vi "sit IO cRIO9113.vi"() -> ()   [LabVIEW 2010]
uses:
  <vilib>/Platform/TimedLoop/XDataNode/XDataNode.xnode
  <vilib>/Platform/TimedLoop/XDataNode/timing_clust.ctl
  <vilib>/Platform/TimedLoop/XDataNode/nitl_modes.ctl
  <vilib>/Platform/TimedLoop/XDataNode/wakeup.ctl
  <vilib>/eio/EIONode/EIONode.xnode
  <vilib>/rvi/eio/nirviEIOImplementation/nirviEIOImplementation.xnode
  <vilib>/rvi/eio/common/nirviEmuClasses.ctl
  <vilib>/rvi/Arithmetic/AddSubMult/XNode/nirviSatArithmetic.xnode
  <vilib>/rvi/eio/common/nirviEmuTemplateMethod_noerrors.vi
  <vilib>/Platform/TimedLoop/XDataNode/XDNodeRunTimeDep.lvlib
panel:
  in  "Velocity Interval (uSec)":u32=200000
  out "Velocity (Counts/Interval)":i32
  out "Acceleration (Counts/Interval)":i32
  out "Position (Counts)":i32
  in  "Position Reset 2":bool
  out "Rudder (Counts)":i32
  in  "Rudder Position Reset":bool
  in  "PWM out 2 (DO 6)":u32[](array[numeric])=[0, 0]
  in  "PWM out 3 (DO 7)":u32[](array[numeric])=[0, 0]
  in  "_PWM In 1 timeout":u32=40000
  out "_PWM In 1 High Time":u32
  out "_PWM In 1 Low Time":u32
  out "_PWM In 0 Low Time":u32
  out "_PWM In 0 High Time":u32
  in  "_PWM In 0 timeout":u32=40000
  in  "_Low Pulse 1":u32
  in  "_High Pulse 1":u32
  in  "_Low Pulse 3":u32
  in  "_High Pulse 3":u32
  in  "_Low Pulse 2":u32
  in  "_High Pulse 2":u32
  in  "PWM out 0 (DO 4)":u32[](array[numeric])=[0, 0]
  in  "PWM out 1 (DO 5)":u32[](array[numeric])=[0, 0]
  out "PWM in 1 (DI 5)":u32[](array[numeric])
  out "PWM in 0 (DI 4)":u32[](array[numeric])
  in  "_Low Pulse 0":u32
  in  "_High Pulse 0":u32
  in  "DO 0":bool
  in  "DO 1":bool
  in  "DO 2":bool
  in  "DO 3":bool
  out "DI 4":bool
  out "DI 5":bool
  in  "Reset":bool
  out "Late? Latched":bool
  in  "Wait Until Cleared":bool=TRUE
  in  "Local Stop 0":bool
  in  "Start 0":bool
  in  "_IRQ bit (0-31)":u8
  in  "Loop Rate (usec)":u32=300
  # "Configuration"
  # "Encoders"
  # "Digital"
  # "PWM"
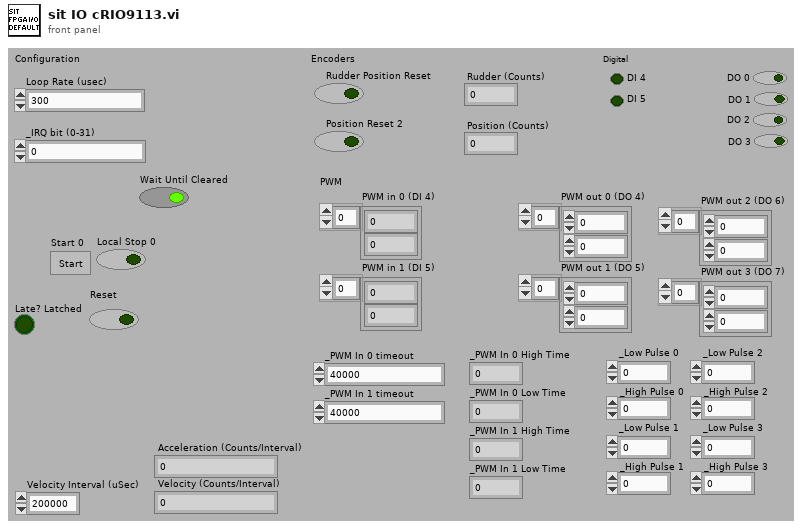
[diagram p1: front panel]
types:
  T1 = typedef "XDNodeRunTimeDep.lvlib/timing_clust.ctl" = cluster{"Expected End [f-1]":u64, "Actual End [f-1]":u64, "Finished Late? [f-1]":bool, "Expected End [i-1]":u64, "Actual End [i-1]":u64, "Finished Late? [i-1]":bool, "Expected Start [i]":u64, "Actual Start [i]":u64, "Expected Start [f]":u64, "Actual Start [f]":u64, "Source Name":string, "Structure Name":string, "Period":i64, "Deadline":i64, "Offset":i64, "Start":i64, "Priority":i32, "Timeout":i32, "Mode":T2, "Wakeup Reason":T3, "Error":errorcluster, "Source Type":string, "Secondary Source Type":string, "Global End Time":u64, "Global Start Time":u64, "Frame Duration":u64, "Iteration Duration":u64, "Assigned CPU":i32, "I/O Scan Engine Mode":u32}
  T2 = typedef "XDNodeRunTimeDep.lvlib/nitl_modes.ctl" = enum32{"No Change", "Process missed periods, maintain original phase", "Discard missed periods, maintain original phase", "Process missed periods, ignore original phase", "Discard missed periods, ignore original phase"}
  T3 = typedef "XDNodeRunTimeDep.lvlib/wakeup.ctl" = enum32{"Normal", "Aborted", "Asynchronous wakeup", "Timing source error", "Timed loop error", "Timeout"}
  T4 = typedef "nirviEmuClasses.ctl" = enum16{"IO Read", "IO Write", "Method", "Property Read", "Property Write"}
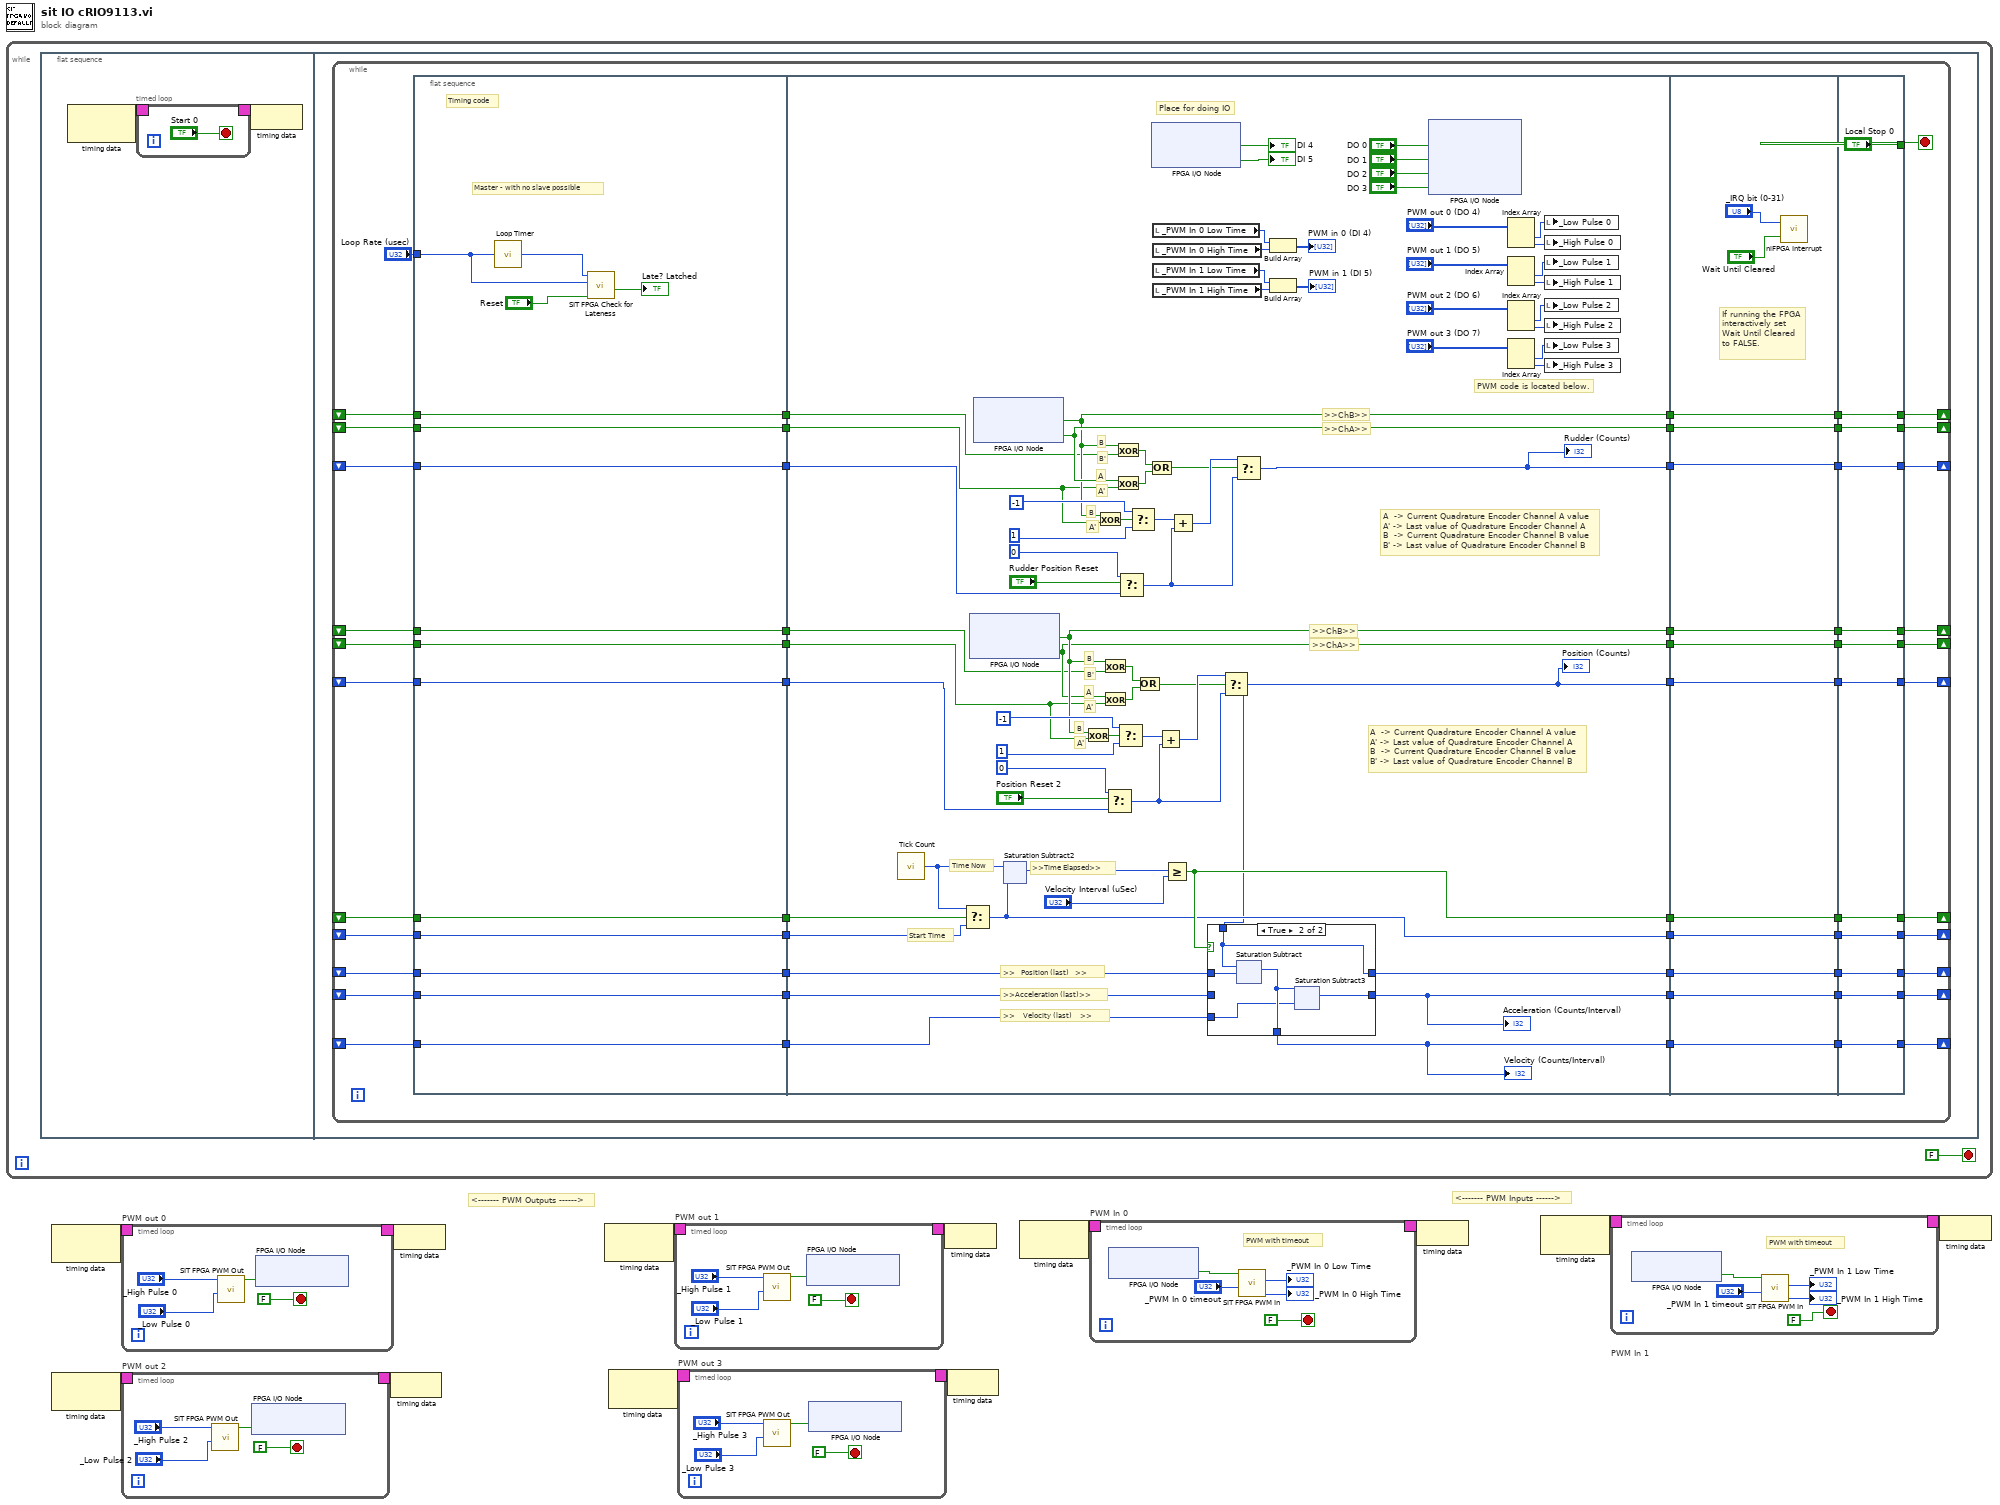
[diagram p0: block diagram]
diagram:
  # "<------- PWM Outputs ------>"
  # "<------- PWM Inputs ------>"
  n1 = while {
    stop <- FALSE stop-if-true
    n2 = flat-sequence {
      frame #0 {
        n3 = node-c288 ("Input Node")() -> (w15:T1)  [unwired: 1 out]
        n4 = timed-loop "initWait" {
          timing: w15 -> [_]
          timing-out: [_] -> w14
          stop <- "Start 0" stop-if-true
        }
        n5 = node-c288 ("Output Node")(w14) -> ()
      }
      frame #1 {
        n6 = while {
          shift-right: [w72] -> _
          shift-left: _ -> [w65]
          shift-right: [w73] -> _
          shift-left: _ -> [w63]
          shift-right: [w69] -> _
          shift-left: _ -> [w61]
          shift-right: [w60] -> _
          shift-left: _ -> [w50]
          shift-right: [w57] -> _
          shift-left: _ -> [w48]
          shift-right: [w54] -> _
          shift-left: _ -> [w46]
          shift-right: [w45] -> _
          shift-left: _ -> [w29]
          shift-right: [w39] -> _
          shift-left: _ -> [w25]
          shift-right: [w42] -> _
          shift-left: _ -> [w27]
          shift-right: [w36] -> _
          shift-left: _ -> [w23]
          shift-right: [w33] -> _
          shift-left: _ -> [w21]
          stop <- w76 stop-if-true
          n7 = flat-sequence {
            tunnel: "Loop Rate (usec)" -> [w78]
            tunnel: [w89] -> w66
            tunnel: w65 -> [w89]
            tunnel: [w88] -> w64
            tunnel: w63 -> [w88]
            tunnel: [w87] -> w62
            tunnel: w61 -> [w87]
            tunnel: [w86] -> w51
            tunnel: w50 -> [w86]
            tunnel: [w85] -> w49
            tunnel: w48 -> [w85]
            tunnel: [w84] -> w47
            tunnel: w46 -> [w84]
            tunnel: [w83] -> w30
            tunnel: w29 -> [w83]
            tunnel: [w82] -> w28
            tunnel: w27 -> [w82]
            tunnel: [w81] -> w26
            tunnel: w25 -> [w81]
            tunnel: [w80] -> w24
            tunnel: w23 -> [w80]
            tunnel: [w79] -> w22
            tunnel: w21 -> [w79]
            tunnel: [w128] -> w74
            tunnel: [w127] -> w70
            tunnel: [w97] -> w67
            tunnel: w66 -> [w126]
            tunnel: w64 -> [w125]
            tunnel: w62 -> [w124]
            tunnel: [w112] -> w58
            tunnel: [w111] -> w55
            tunnel: [w96] -> w52
            tunnel: w51 -> [w110]
            tunnel: w49 -> [w109]
            tunnel: w47 -> [w108]
            tunnel: [w105] -> w43
            tunnel: [w104] -> w40
            tunnel: [w103] -> w37
            tunnel: [w94] -> w34
            tunnel: [w93] -> w31
            tunnel: w30 -> [w102]
            tunnel: w28 -> [w101]
            tunnel: w26 -> [w100]
            tunnel: w24 -> [w99]
            tunnel: w22 -> [w98]
            tunnel: [w386] -> w75
            tunnel: w74 -> [w386]
            tunnel: [w385] -> w71
            tunnel: w70 -> [w385]
            tunnel: [w384] -> w68
            tunnel: w67 -> [w384]
            tunnel: [w383] -> w59
            tunnel: w58 -> [w383]
            tunnel: [w382] -> w56
            tunnel: w55 -> [w382]
            tunnel: [w381] -> w53
            tunnel: w52 -> [w381]
            tunnel: [w380] -> w44
            tunnel: w43 -> [w380]
            tunnel: [w379] -> w41
            tunnel: w40 -> [w379]
            tunnel: [w378] -> w38
            tunnel: w37 -> [w378]
            tunnel: [w377] -> w35
            tunnel: w34 -> [w377]
            tunnel: [w376] -> w32
            tunnel: w31 -> [w376]
            tunnel: ["Local Stop 0"] -> w76
            tunnel: [w399] -> w73
            tunnel: w75 -> [w399]
            tunnel: [w398] -> w72
            tunnel: w71 -> [w398]
            tunnel: [w397] -> w69
            tunnel: w68 -> [w397]
            tunnel: [w396] -> w60
            tunnel: w59 -> [w396]
            tunnel: [w395] -> w57
            tunnel: w56 -> [w395]
            tunnel: [w394] -> w54
            tunnel: w53 -> [w394]
            tunnel: [w393] -> w45
            tunnel: w44 -> [w393]
            tunnel: [w392] -> w42
            tunnel: w41 -> [w392]
            tunnel: [w391] -> w39
            tunnel: w38 -> [w391]
            tunnel: [w390] -> w36
            tunnel: w35 -> [w390]
            tunnel: [w389] -> w33
            tunnel: w32 -> [w389]
            frame #0 {
              # "Master - with no slave possible"
              # "Timing code"
              n8 = call "Loop Timer"("Count(uSec)"=w78) -> ("Tick Count(uSec)"=w91:u32)
              n9 = call <vilib>:"SIT FPGA Check for Lateness.vi"("Reset"="Reset", "Loop Rate (usec)"=w78, "Tick Count(uSec)"=w91) -> ("Late? Latched"=→"Late? Latched":bool)  [unwired: 1 in, 7 out]
            }
            frame #1 {
              # ">>Acceleration (last)>>"
              # "Start Time"
              # ">>    Velocity (last)    >>"
              # ">>   Position (last)   >>"
              # "Time Now"
              # ">>Time Elapsed>>"
              # "A  -> Current Quadrature Encoder Channel A value\nA' -> Last value of Quadrature Encoder Channel A\nB  -> Current Quadrature Encoder Channel B value\nB' -> Last value of Quadrature Encoder Channel B"
              # "A'"
              # "B"
              # "A'"
              # "A"
              # "B'"
              # "B"
              # ">>ChB>>"
              # ">>ChA>>"
              # "A  -> Current Quadrature Encoder Channel A value\nA' -> Last value of Quadrature Encoder Channel A\nB  -> Current Quadrature Encoder Channel B value\nB' -> Last value of Quadrature Encoder Channel B"
              # "A'"
              # "B"
              # "A'"
              # "A"
              # "B'"
              # "B"
              # ">>ChB>>"
              # ">>ChA>>"
              # "PWM code is located below."
              # "Place for doing IO"
              n10 = call "Tick Count"() -> ("Tick Count(uSec)"=w106:u32)
              n11 = Select(t=w106, s=w102, f=w101) -> (s? t:f=w104:u32)
              n12 = xnode "FPGA I/O Node"() -> ("NI 9411/DI3"=w112:bool, "NI 9411/DI2"=w111:bool)  [unwired: 2 in, 2 out]
              n13 = xnode "FPGA I/O Node"() -> ("NI 9411/DI1"=w127:bool, "NI 9411/DI0"=w128:bool)  [unwired: 2 in, 2 out]
              n14 = xnode ("Saturation Subtract2")("x"=w106, "y"=w104) -> ("x-y"=w95:u32)
              n15 = Exclusive Or(1:w109, 2:w112) -> (0:w114:bool)
              n16 = Exclusive Or(1:w125, 2:w127) -> (0:w130:bool)
              n17 = Exclusive Or(1:w110, 2:w112) -> (0:w115:bool)
              n18 = Exclusive Or(1:w109, 2:w111) -> (0:w116:bool)
              n19 = Select(t=0 ("32 bit"), s="Position Reset 2", f=w108) -> (s? t:f=w121:i32)
              n20 = Exclusive Or(1:w126, 2:w127) -> (0:w131:bool)
              n21 = Exclusive Or(1:w125, 2:w128) -> (0:w132:bool)
              n22 = Select(t=-1 ("32 bit"), s=w114, f=1 ("32 bit")) -> (s? t:f=w119:i32)
              n23 = Select(t=0 ("32 bit"), s="Rudder Position Reset", f=w124) -> (s? t:f=w137:i32)
              n24 = Select(t=-1 ("32 bit"), s=w130, f=1 ("32 bit")) -> (s? t:f=w135:i32)
              n25 = Or(x=w115, y=w116) -> (x .or. y?=w113:bool)
              n26 = Or(x=w131, y=w132) -> (x .or. y?=w129:bool)
              n27 = xnode "FPGA I/O Node"() -> ("NI 9411/DI4"=→"DI 4":bool, "NI 9411/DI5"=→"DI 5":bool)  [unwired: 2 in, 2 out]
              n28 = local read "_PWM In 0 Low Time"() -> (w156:u32)
              n29 = local read "_PWM In 0 High Time"() -> (w157:u32)
              n30 = local read "_PWM In 1 Low Time"() -> (w152:u32)
              n31 = local read "_PWM In 1 High Time"() -> (w153:u32)
              n32 = Add(x=w119, y=w121) -> (x+y=w123:i32)
              n33 = Greater Or Equal?(x=w95, y="Velocity Interval (uSec)") -> (x >= y?=w105:bool)
              n34 = Add(x=w135, y=w137) -> (x+y=w139:i32)
              n35 = Select(t=w123, s=w113, f=w121) -> (s? t:f=w96:i32)
              "Position (Counts)" <- w96
              n36 = case shown="True" w105 {
                tunnel: w96 -> [_ w177]
                tunnel: w100 -> [w174 w181]
                tunnel: [w176 w180] -> w93
                tunnel: w98 -> [w176 w179]
                tunnel: [w175 w178] -> w94
                tunnel: w99 -> [w175 _]
                tunnel: [w174 w177] -> w103
                frame False {
                }
                frame True {
                  n37 = xnode ("Saturation Subtract")("x"=w177, "y"=w181) -> ("x-y"=w180:i32)
                  n38 = xnode ("Saturation Subtract3")("x"=w180, "y"=w179) -> ("x-y"=w178:i32)
                }
              }
              "Acceleration (Counts/Interval)" <- w94
              "Velocity (Counts/Interval)" <- w93
              n39 = Select(t=w139, s=w129, f=w137) -> (s? t:f=w97:i32)
              "Rudder (Counts)" <- w97
              n40 = Build Array(w156, w157) -> (→"PWM in 0 (DI 4)":u32[])
              n41 = Build Array(w152, w153) -> (→"PWM in 1 (DI 5)":u32[])
              n42 = xnode "FPGA I/O Node"("NI 9474/DO0"="DO 0", "NI 9474/DO1"="DO 1", "NI 9474/DO2"="DO 2", "NI 9474/DO3"="DO 3") -> ()  [unwired: 4 in, 4 out]
              n43 = Index Array(array="PWM out 0 (DO 4)") -> (element #1=w150:u32, element #2=w151:u32)  [unwired: 2 in]
              n44 = Index Array(array="PWM out 1 (DO 5)") -> (element #1=w148:u32, element #2=w149:u32)  [unwired: 2 in]
              n45 = Index Array(array="PWM out 2 (DO 6)") -> (element #1=w141:u32, element #2=w140:u32)  [unwired: 2 in]
              n46 = Index Array(array="PWM out 3 (DO 7)") -> (element #1=w143:u32, element #2=w142:u32)  [unwired: 2 in]
              n47 = local write "_Low Pulse 0"(w150) -> ()
              n48 = local write "_High Pulse 0"(w151) -> ()
              n49 = local write "_Low Pulse 1"(w148) -> ()
              n50 = local write "_High Pulse 1"(w149) -> ()
              n51 = local write "_Low Pulse 2"(w141) -> ()
              n52 = local write "_High Pulse 2"(w140) -> ()
              n53 = local write "_Low Pulse 3"(w143) -> ()
              n54 = local write "_High Pulse 3"(w142) -> ()
            }
            frame #2 {
              # "If running the FPGA interactively set Wait Until Cleared to FALSE."
              n55 = call <vilib>:"niFPGA Interrupt.vi"("Wait Until Cleared"="Wait Until Cleared", "IRQ Number"="_IRQ bit (0-31)") -> ()  [unwired: 1 in]
            }
            frame #3 {
            }
          }
        }
      }
    }
  }
  n56 = node-c288() -> (w12:T1)  [unwired: 1 out]
  n57 = node-c288() -> (w10:T1)  [unwired: 1 out]
  n58 = timed-loop "PWM out 0" {
    timing: w12 -> [_]
    timing-out: [_] -> w11
    stop <- FALSE stop-if-true
    n59 = call <vilib>:"SIT FPGA PWM Out.vi"("_Low Time"="_Low Pulse 0", "_High Time"="_High Pulse 0") -> ("Output"=w403:bool)  [unwired: 1 in, 8 out]
    n60 = xnode "FPGA I/O Node"("NI 9474/DO4"=w403) -> ()  [unwired: 1 in, 1 out]
  }
  n61 = timed-loop "PWM out 2" {
    timing: w10 -> [_]
    timing-out: [_] -> w9
    stop <- FALSE stop-if-true
    n62 = call <vilib>:"SIT FPGA PWM Out.vi"("_Low Time"="_Low Pulse 2", "_High Time"="_High Pulse 2") -> ("Output"=w420:bool)  [unwired: 1 in, 8 out]
    n63 = xnode "FPGA I/O Node"("NI 9474/DO6"=w420) -> ()  [unwired: 1 in, 1 out]
  }
  n64 = node-c288(w9) -> ()
  n65 = node-c288(w11) -> ()
  n66 = node-c288() -> (w8:T1)  [unwired: 1 out]
  n67 = node-c288() -> (w6:T1)  [unwired: 1 out]
  n68 = timed-loop "PWM out 1" {
    timing: w8 -> [_]
    timing-out: [_] -> w7
    stop <- FALSE stop-if-true
    n69 = call <vilib>:"SIT FPGA PWM Out.vi"("_Low Time"="_Low Pulse 1", "_High Time"="_High Pulse 1") -> ("Output"=w435:bool)  [unwired: 1 in, 8 out]
    n70 = xnode "FPGA I/O Node"("NI 9474/DO5"=w435) -> ()  [unwired: 1 in, 1 out]
  }
  n71 = timed-loop "PWM out 3" {
    timing: w6 -> [_]
    timing-out: [_] -> w5
    stop <- FALSE stop-if-true
    n72 = call <vilib>:"SIT FPGA PWM Out.vi"("_Low Time"="_Low Pulse 3", "_High Time"="_High Pulse 3") -> ("Output"=w455:bool)  [unwired: 1 in, 8 out]
    n73 = xnode "FPGA I/O Node"("NI 9474/DO7"=w455) -> ()  [unwired: 1 in, 1 out]
  }
  n74 = node-c288(w7) -> ()
  n75 = node-c288(w5) -> ()
  n76 = node-c288() -> (w4:T1)  [unwired: 1 out]
  n77 = timed-loop "PWM In 0" {
    timing: w4 -> [_]
    timing-out: [_] -> w3
    stop <- FALSE stop-if-true
    # "PWM with timeout"
    n78 = xnode "FPGA I/O Node"() -> ("NI 9411/DI4"=w472:bool)  [unwired: 1 in, 1 out]
    n79 = call <vilib>:"SIT FPGA PWM In.vi"("Time Out"="_PWM In 0 timeout", "Value"=w472) -> ("High time"=→"_PWM In 0 High Time":u32, "Low Time"=→"_PWM In 0 Low Time":u32)  [unwired: 8 out]
  }
  n80 = node-c288(w3) -> ()
  n81 = node-c288() -> (w2:T1)  [unwired: 1 out]
  n82 = timed-loop "PWM In 1" {
    timing: w2 -> [_]
    timing-out: [_] -> w1
    stop <- FALSE stop-if-true
    # "PWM with timeout"
    n83 = xnode "FPGA I/O Node"() -> ("NI 9411/DI5"=w498:bool)  [unwired: 1 in, 1 out]
    n84 = call <vilib>:"SIT FPGA PWM In.vi"("Time Out"="_PWM In 1 timeout", "Value"=w498) -> ("High time"=→"_PWM In 1 High Time":u32, "Low Time"=→"_PWM In 1 Low Time":u32)  [unwired: 8 out]
  }
  n85 = node-c288(w1) -> ()
